vi "Generate_Waveform_from_File.vi"() -> ()   [LabVIEW 2020]
uses:
  <instrlib>/niFgen/niFgen.llb/niFgen Output Mode.ctl
  <vilib>/Utility/file.llb/Read Delimited Spreadsheet (DBL).vi
  <instrlib>/niFgen/niFgen.llb/niFgen Create Waveform (DBL).vi
panel:
  in  "Stop":bool
  in  "Sample Rate":dbl=50000000.0 format="%.2p"
  in  "FGEN Resource Name 2":refnum<k15>="FGEN2" caption="FGEN Resource Name"
  in  "file to run":path=path "C:/Users/Puja/Desktop/Labview(PC)/Input_Signal/Sine_wave_data_without_time/data1_w1_NT_1per.txt"
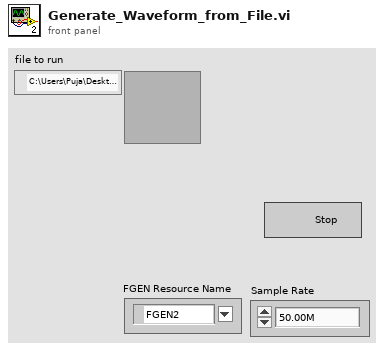
[diagram p1: front panel]
types:
  T1 = typedef "niFgen Output Mode.ctl" = u32
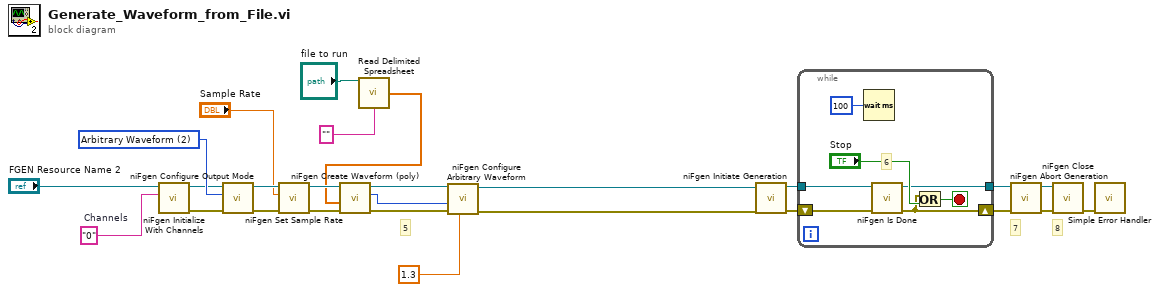
[diagram p0: block diagram]
diagram:
  w20 = "0"  # Channels
  w24 = T1 2 items=["Standard Function", "Frequency List", "Arbitrary Waveform", "Arbitrary Sequence", "Script"] ("output mode")
  # "8"
  # "7"
  # "5"
  n1 = call <instrlib>:"niFgen Initialize With Channels.vi"("Channel Name"=w20, "Resource Name"="FGEN Resource Name 2") -> ("error out"=w23:errorcluster, "Instrument Handle Out"=w22:refnum<k15>)  [unwired: 8 in]
  n2 = call <instrlib>:"niFgen Configure Output Mode.vi"("error in (no error)"=w23, "Output Mode (default: 0=Standard Function)"=w24, "Instrument Handle"=w22) -> ("error out"=w18:errorcluster, "Instrument Handle Out"=w19:refnum<k15>)  [unwired: 6 in]
  n3 = call <instrlib>:"niFgen Set Sample Rate.vi"("error in (no error)"=w18, "Sample Rate (Samp/s)"="Sample Rate", "Instrument Handle"=w19) -> ("error out"=w15:errorcluster, "Instrument Handle Out"=w16:refnum<k15>)  [unwired: 7 in]
  n4 = call-poly <vilib>:"Read Delimited Spreadsheet.vi"("file path (dialog if empty)"="file to run", "delimiter (\\t)"="") -> ("first row"=w7:dbl[])  [unwired: 8 in, 5 out]
  n5 = call-poly <instrlib>:"niFgen Create Waveform (poly).vi"("error in (no error)"=w15, "Waveform Data Array"=w7, "Instrument Handle"=w16) -> ("error out"=w5:errorcluster, "Waveform Handle"=w1:i32, "Instrument Handle Out"=w6:refnum<k15>)  [unwired: 6 in]
  n6 = call <instrlib>:"niFgen Configure Arbitrary Waveform.vi"("Gain"=1.3, "error in (no error)"=w5, "Waveform Handle"=w1, "Instrument Handle"=w6) -> ("error out"=w4:errorcluster, "Instrument Handle Out"=w3:refnum<k15>)  [unwired: 6 in]
  n7 = call <instrlib>:"niFgen Initiate Generation.vi"("error in (no error)"=w4, "Instrument Handle"=w3) -> ("error out"=w13:errorcluster, "Instrument Handle Out"=w12:refnum<k15>)  [unwired: 8 in]
  n8 = while {
    tunnel: w12 -> [w30]
    tunnel: [w27] -> w10
    shift-right: [w28] -> w11
    shift-left: w13 -> [w29]
    stop <- w33 stop-if-true
    # "6"
    n9 = Wait (ms)(milliseconds to wait=u32 100 ("millisecond multiple")) -> ()  [unwired: 1 out]
    n10 = call <instrlib>:"niFgen Is Done.vi"("error in (no error)"=w29, "Instrument Handle"=w30) -> ("error out"=w28:errorcluster, "Instrument Handle Out"=w27:refnum<k15>)  [unwired: 7 in, 1 out]
    n11 = Or(x=w28, y="Stop") -> (x .or. y?=w33:bool)
  }
  n12 = call <instrlib>:"niFgen Abort Generation.vi"("error in (no error)"=w11, "Instrument Handle"=w10) -> ("error out"=w9:errorcluster, "Instrument Handle Out"=w8:refnum<k15>)  [unwired: 8 in]
  n13 = call <instrlib>:"niFgen Close.vi"("error in (no error)"=w9, "Instrument Handle"=w8) -> ("error out"=w14:errorcluster)  [unwired: 9 in]
  n14 = call <vilib>:"Simple Error Handler.vi"("error in (no error)"=w14) -> ()  [unwired: 4 in, 5 out]
